vi "Project Items - Get Names.vi"(8 "Error In":errorcluster, 11 "Project Items":refnum<vi>[](array[refnum])) -> (0 "Error Out":errorcluster, 3 "Project Item Names":string[](array[string]))   [LabVIEW 2022 SP3]
doc: "<add documentation here>"
panel:
  # "Development\nControls or indicators that are useful for development or testing, but which are not outputs of the VI."
  # "Input\nInputs to the VI"
  # "Output\nOutputs of the VI"
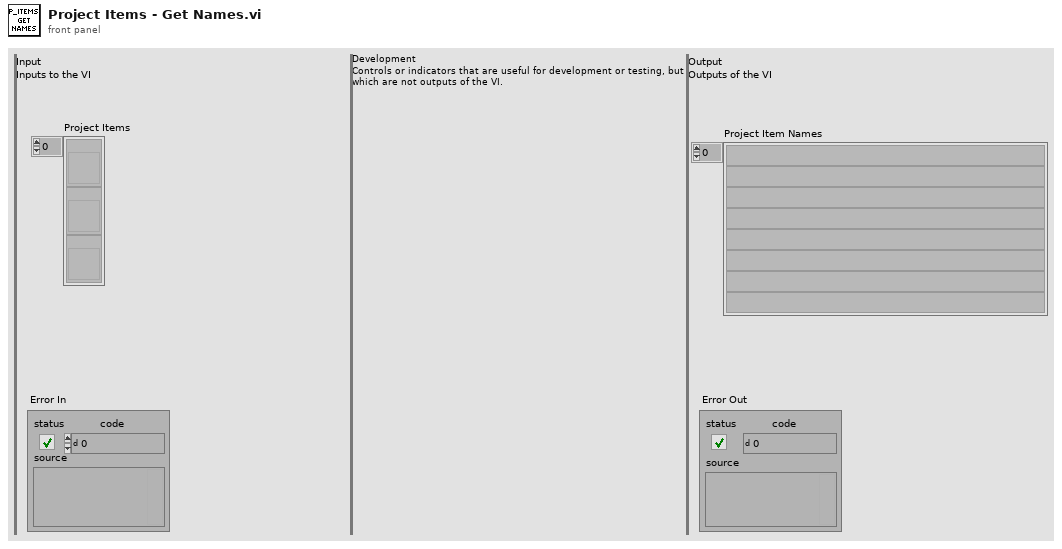
[diagram p1: front panel]
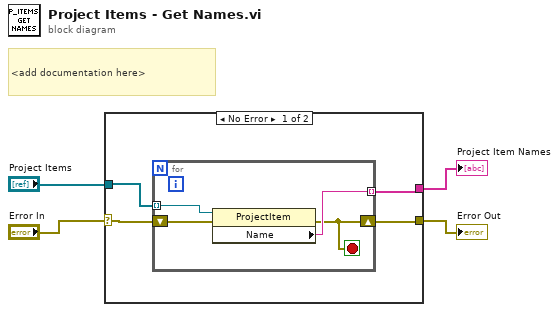
[diagram p0: block diagram]
diagram:
  # "<add documentation here>"
  n1 = case shown="No Error" "Error In" {
    selector: "Error In" -> [w8 w13]
    tunnel: [w6 w13] -> w3
    tunnel: "Project Items" -> [w7 _]
    tunnel: [w5 _] -> w1
    frame No Error {
      n2 = for {
        tunnel: w7 -> [w12] mode=indexing
        shift-right: [w9] -> w6
        shift-left: w8 -> [w11]
        tunnel: [w10] -> w5 mode=indexing
        stop <- w9 stop-if-true
        n3 = property class="ProjectItem"(reference=w12, error in=w11) -> (error out=w9:errorcluster, "Name"=w10:string)  [unwired: 1 out]
      }
    }
    frame Error {
    }
  }
  "Error Out" <- w3
  "Project Item Names" <- w1
